vi "Read Token.vi"(9 "Termination":string, 10 "Token":string, 11 "Status In":string) -> (1 "Parsed Value":string, 3 "Status out":string)   [LabVIEW 2018, in "Kronos.lvlib" / "Kronos.lvclass"]
uses:
  Kronos.lvclass
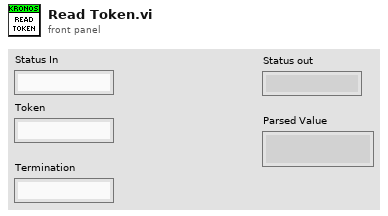
[diagram p1: front panel]
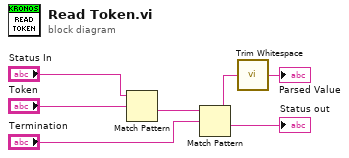
[diagram p0: block diagram]
diagram:
  n1 = Match Pattern(string="Status In", regular expression="Token") -> (after substring=w5:string)  [unwired: 1 in, 3 out]
  n2 = Match Pattern(string=w5, regular expression="Termination") -> (before substring=w2:string, after substring=→"Status out":string)  [unwired: 1 in, 2 out]
  n3 = call <vilib>:"Trim Whitespace.vi"("string"=w2) -> ("trimmed string"=→"Parsed Value":string)  [unwired: 1 in]
